vi "AlliGator Save Hot Pixel Mask Image.vi"(8 "error in (no error)":errorcluster, 9 "Saved Image File Format":T2, 10 "File Path in":path, 11 "Image Refnum in":T1) -> (0 "Error Out":errorcluster, 2 "File Path out":path)   [LabVIEW 2021, in "AlliGator Files.lvlib"]
doc: "Saves image as 8-bit binary Mask Image."
uses:
  Image/Image Save File Format.ctl
  <vilib>/vision/Image Controls.llb/IMAQ Image.ctl
  AlliGator Files.lvlib
  Image/Image.lvlib
panel:
  # "see the AlliGator License on the block diagram (Ctrl+E or Window:Show Block Diagram)"
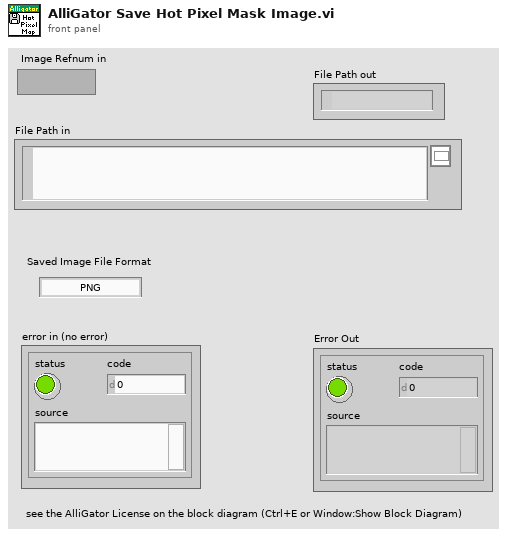
[diagram p1: front panel]
types:
  T1 = typedef "IMAQ Image.ctl" = refnum<image>
  T2 = typedef "Image.lvlib/Image Save File Format.ctl" = enum16{"PNG", "JPEG", "BMP"}
  T3 = typedef "Image Type" = u32
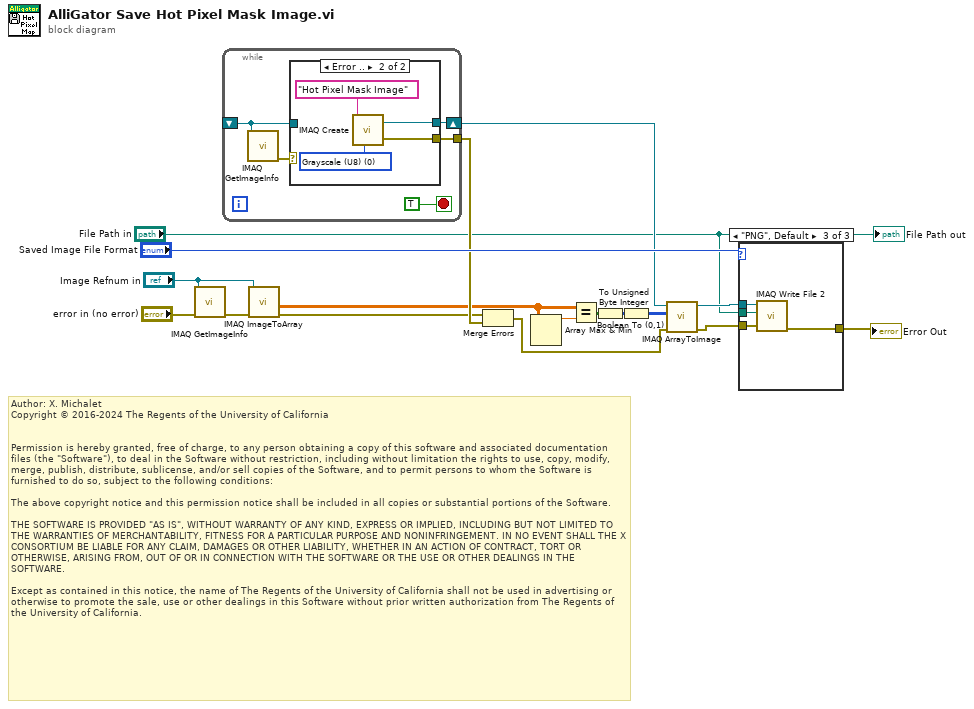
[diagram p0: block diagram]
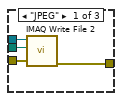
[diagram p2: hidden frame]
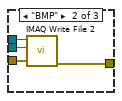
[diagram p3: hidden frame]
diagram:
  # "Author: X. Michalet\nCopyright © 2016-2024 The Regents of the University of California\n \n\nPermission is hereby granted, free of charge, to any person obtaining a copy of this software and associated documentation files (the \"Software\"), to deal in the Software without restriction, including without limitation the rights to use, copy, modify, merge, publish, distribute, sublicense, and/or sell copies of the Software, and to permit persons to whom the Software is furnished to do so, subject to the following conditions:\n\nThe above copyright notice and this permission notice shall be included in all copies or substantial portions of the Software.\n\nTHE SOFTWARE IS PROVIDED \"AS IS\", WITHOUT WARRANTY OF ANY KIND, EXPRESS OR IMPLIED, INCLUDING BUT NOT LIMITED TO THE WARRANTIES OF MERCHANTABILITY, FITNESS FOR A PARTICULAR PURPOSE AND NONINFRINGEMENT. IN NO EVENT SHALL THE X CONSORTIUM BE LIABLE FOR ANY CLAIM, DAMAGES OR OTHER LIABILITY, WHETHER IN AN ACTION OF CONTRACT, TORT OR OTHERWISE, ARISING FROM, OUT OF OR IN CONNECTION WITH THE SOFTWARE OR THE USE OR OTHER DEALINGS IN THE SOFTWARE.\n\nExcept as contained in this notice, the name of The Regents of the University of California shall not be used in advertising or otherwise to promote the sale, use or other dealings in this Software without prior written authorization from The Regents of the University of California."
  n1 = call "IMAQ GetImageInfo"("error in (no error)"="error in (no error)", "Image"="Image Refnum in") -> ("error out"=w15:errorcluster)  [unwired: 2 in, 7 out]
  n2 = while {
    shift-right: [w21] -> w9
    shift-left: _ -> [w20]
    tunnel: [w19] -> w12
    stop <- TRUE stop-if-true
    n3 = call "IMAQ GetImageInfo"("Image"=w20) -> ("error out"=w18:errorcluster)  [unwired: 3 in, 7 out]
    n4 = case shown="Error .." w18 {
      selector: w18 -> [w23 _]
      tunnel: [w24 w27] -> w21
      tunnel: w20 -> [w24 _]
      tunnel: [w23 w26] -> w19
      frame No Error {
      }
      frame Error {
        w25 = T3 0 items=["Grayscale (U8)", "Grayscale (I16)", "Grayscale (SGL)", "Complex (CSG)", "RGB (U32)", "HSL (U32)", "RGB (U64)", "Grayscale (U16)"] ("Image Type")
        n5 = call "IMAQ Create"("Image Name"="Hot Pixel Mask Image", "Image Type"=w25) -> ("New Image"=w27:T1, "error out"=w26:errorcluster)  [unwired: 3 in]
      }
    }
  }
  n6 = call "IMAQ ImageToArray"("error in (no error)"=w15, "Image"="Image Refnum in") -> ("Image Pixels (Float)"=w4:sgl[][], "error out"=w10:errorcluster)  [unwired: 2 in, 3 out]
  n7 = Merge Errors(w10, w12) -> (w11:errorcluster)
  n8 = Array Max & Min(array=w4) -> (max value=w5:sgl)  [unwired: 3 out]
  n9 = Equal?(x=w4, y=w5) -> (x = y?=w3:bool[][])
  n10 = Boolean To (0,1)(Boolean=w3) -> (0, 1=w2:i16[][])
  n11 = To Unsigned Byte Integer(number=w2) -> (unsigned 8bit integer=w1:u8[][])
  n12 = call "IMAQ ArrayToImage"("error in (no error)"=w11, "Image Pixels (U8)"=w1, "Image"=w9) -> ("error out"=w8:errorcluster, "Image Out"=w7:T1)  [unwired: 7 in]
  n13 = case shown="\"PNG\", Default" "Saved Image File Format" {
    tunnel: w8 -> [w32 w36 w40]
    tunnel: w7 -> [w31 w35 w39]
    tunnel: [w30 w34 w38] -> w16
    tunnel: "File Path in" -> [w29 w33 w37]
    frame "JPEG" {
      n14 = call-poly "IMAQ Write File 2"("error in (no error)"=w32, "File Path"=w29, "Image"=w31) -> ("error out"=w30:errorcluster)  [unwired: 7 in, 1 out]
    }
    frame "BMP" {
      n15 = call-poly "IMAQ Write File 2"("error in (no error)"=w36, "File Path"=w33, "Image"=w35) -> ("error out"=w34:errorcluster)  [unwired: 7 in, 1 out]
    }
    frame "PNG", Default {
      n16 = call-poly "IMAQ Write File 2"("error in (no error)"=w40, "File Path"=w37, "Image"=w39) -> ("error out"=w38:errorcluster)  [unwired: 7 in, 1 out]
    }
  }
  "Error Out" <- w16
  "File Path out" <- "File Path in"
